vi "Read NeadleValve.vi"(11 "Stand in":refnum<class "Stand.lvclass">) -> (1 "NeadleValve_2":refnum<class "NeedleValve.lvclass">, 2 "NeedleValve_1":refnum<class "NeedleValve.lvclass">)   [LabVIEW 2019, in "Stand.lvclass"]
uses:
  Stand.lvclass
  NeedleValve_class/NeedleValve.lvclass
  Stand.lvclass/Stand.ctl
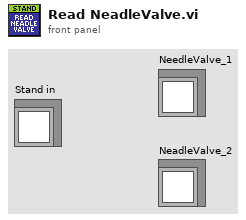
[diagram p1: front panel]
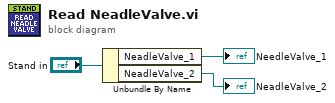
[diagram p0: block diagram]
diagram:
  n1 = Unbundle By Name("Stand in") -> ("NeadleValve_1"=→"NeedleValve_1":refnum<class "NeedleValve.lvclass">, "NeadleValve_2"=→"NeadleValve_2":refnum<class "NeedleValve.lvclass">)
